vi "convert_format.vi"(10 "maximum bit depth":i8=16, 11 "values to be written":T1) -> (2 "data":u64)   [LabVIEW 2010]
uses:
  common_typedefs/channels_cluster.ctl
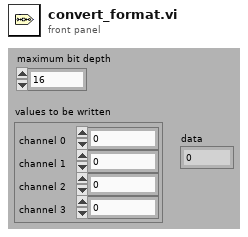
[diagram p1: front panel]
types:
  T1 = typedef "channels_cluster.ctl" = cluster{"channel 0":u32, "channel 1":u32, "channel 2":u32, "channel 3":u32}
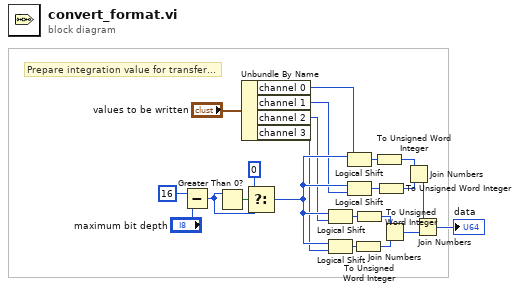
[diagram p0: block diagram]
diagram:
  # "Prepare integration value for transfer..."
  n1 = Subtract(x=i8 16, y="maximum bit depth") -> (x-y=w18:i8)
  n2 = Greater Than 0?(x=w18) -> (x > 0?=w17:bool)
  n3 = Unbundle By Name("values to be written") -> ("channel 0"=w15:u32, "channel 1"=w14:u32, "channel 2"=w13:u32, "channel 3"=w12:u32)
  n4 = Select(t=i8 0 ("f"), s=w17, f=w18) -> (s? t:f=w16:i8)
  n5 = Logical Shift(y=w16, x=w13) -> (x << y=w11:u32)
  n6 = Logical Shift(y=w16, x=w12) -> (x << y=w10:u32)
  n7 = Logical Shift(y=w16, x=w15) -> (x << y=w9:u32)
  n8 = Logical Shift(y=w16, x=w14) -> (x << y=w8:u32)
  n9 = To Unsigned Word Integer(number=w10) -> (unsigned 16bit integer=w6:u16)
  n10 = To Unsigned Word Integer(number=w11) -> (unsigned 16bit integer=w5:u16)
  n11 = To Unsigned Word Integer(number=w9) -> (unsigned 16bit integer=w2:u16)
  n12 = To Unsigned Word Integer(number=w8) -> (unsigned 16bit integer=w7:u16)
  n13 = Join Numbers(hi=w5, lo=w6) -> ((hi.lo)=w4:u32)
  n14 = Join Numbers(hi=w2, lo=w7) -> ((hi.lo)=w3:u32)
  n15 = Join Numbers(hi=w3, lo=w4) -> ((hi.lo)=→"data":u64)
